vi "Remove Multiple Wheels from Steering Frame by Name.vi"(8 "error in (no error)":errorcluster, 10 "wheel names":string[](array[string]), 11 "steering frame in":refnum<class "NI_Robotics_Steering Frame.lvclass">) -> (0 "error out":errorcluster, 1 "found?":bool[](array[boolean]), 2 "removed wheels":refnum<class "NI_Robotics_Wheel.lvclass">[](array[class]), 3 "steering frame out":refnum<class "NI_Robotics_Steering Frame.lvclass">, 4 "frame angles (rad)":dbl[](array[numeric]), 5 "y positions":dbl[](array[numeric]), 7 "x positions":dbl[](array[numeric]))   [LabVIEW 2017, in "NI_Robotics_Steering Frame.lvclass"]
doc: "Removes the wheel or wheels you specify from <B>steering frame in</B>. You must manually select the polymorphic instance to use."
uses:
  <vilib>/robotics/Steering/Steering Frame/NI_Robotics_Steering Frame.lvclass
  <vilib>/robotics/Steering/Wheel/NI_Robotics_Wheel.lvclass
  <vilib>/robotics/Steering/Steering Frame/NI_Robotics_Steering Frame.lvclass/NI_Robotics_Steering Frame.ctl
  <vilib>/robotics/Steering/Wheel/NI_Robotics_Wheel.lvclass/NI_Robotics_Wheel.ctl
  <vilib>/robotics/Steering/Wheel/Get Wheel Name.vi
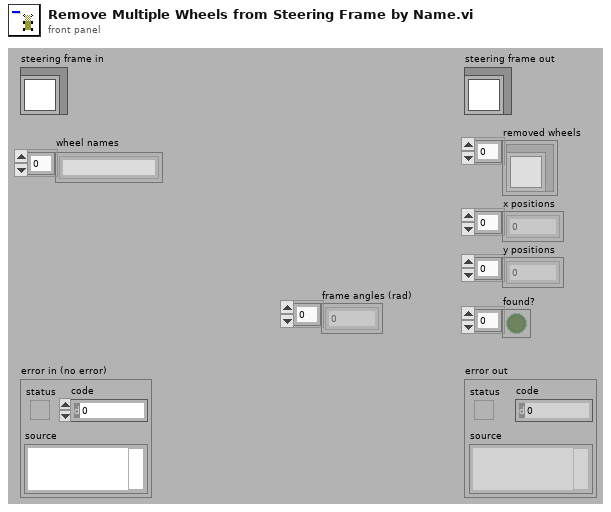
[diagram p1: front panel]
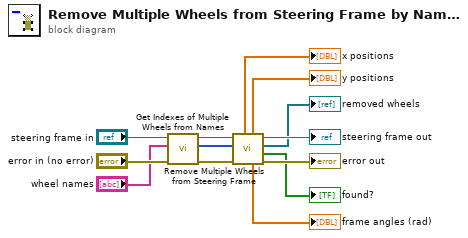
[diagram p0: block diagram]
diagram:
  n1 = call <vilib>:"Get Indexes of Multiple Wheels from Names.vi"("error in (no error)"="error in (no error)", "wheel names"="wheel names", "steering frame in"="steering frame in") -> ("error out"=w9:errorcluster, "indexes"=w8:i32[], "steering frame out"=w10:refnum<class "NI_Robotics_Steering Frame.lvclass">)  [unwired: 5 in, 1 out]
  n2 = call <vilib>:"Remove Multiple Wheels from Steering Frame.vi"("error in (no error)"=w9, "wheel indexes"=w8, "steering frame in"=w10) -> ("error out"=→"error out":errorcluster, "found?"=→"found?":bool[], "removed wheels"=→"removed wheels":refnum<class "NI_Robotics_Wheel.lvclass">[], "steering frame out"=→"steering frame out":refnum<class "NI_Robotics_Steering Frame.lvclass">, "frame angles (rad)"=→"frame angles (rad)":dbl[], "y positions"=→"y positions":dbl[], "x positions"=→"x positions":dbl[])  [unwired: 2 in]
